vi "Experiment with Waveform Generation.vi"(6 "Default Values":T1={"X-Voltage (Default)"=10.0, "Y-Voltage (Default)"=10.0, "Pockels Voltage (Default)"=0.0, "GATE State (Default)"=FALSE}, 7 "Stim Points Array IN":T5[](array[typedef]), 8 "Trigger Parameters":T2, 9 "Sampling Rates":T3, 10 "Group Parameters":T4) -> (0 "Group Duration (Seconds)":dbl, 1 "Gate Wavefprm (digital)":digitalwaveform(waveform)={"t0"=timestamp(0 s since 1904-01-01), "dt"=1.0, "Y"={"transitions"=[], "data"=[]}}, 2 "XY Waveform":waveform(dbl)[](array[waveform]), 3 "Pockels Waveform":waveform(dbl), 4 "Total Protocol Time (s)":dbl, 5 "Stim Waveform Graph":waveform(dbl)[](array[waveform]))   [LabVIEW 2012]
uses:
  Custom Controls and Typedefs/Stim Waveform Parameters.ctl
  Custom Controls and Typedefs/GroupParameters_Cluster.ctl
  Custom Controls and Typedefs/SamplingRatesCluster.ctl
  Custom Controls and Typedefs/TriggerParameters_Cluster.ctl
  Custom Controls and Typedefs/SciScan System Information Cluster.ctl
  GFG/GFGbooleanGet.vi
  GFG/GFGstringGet.vi
  <vilib>/Waveform/DWDTOps.llb/DWDT Boolean Array to Digital.vi
  <vilib>/Utility/config.llb/Read Key (Double).vi
  GFG/GFGnumericGet.vi
  GFG/GFG library.lvlib
  <vilib>/Utility/config.llb/NI_LVConfig.lvlib
panel:
  out "error out":errorcluster
  in  "error in (no error)":errorcluster
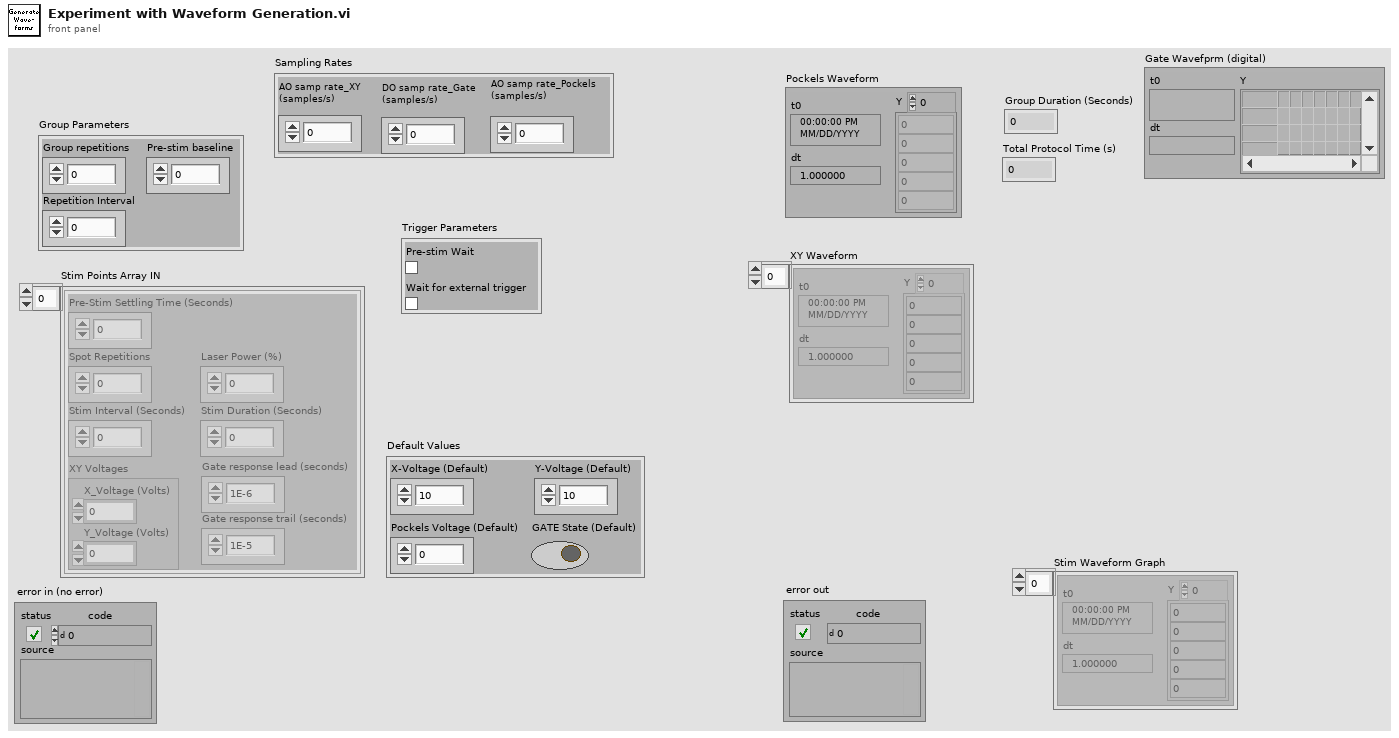
[diagram p1: front panel]
types:
  T1 = cluster{"X-Voltage (Default)":dbl, "Y-Voltage (Default)":dbl, "Pockels Voltage (Default)":dbl, "GATE State (Default)":bool}
  T2 = typedef "TriggerParameters_Cluster.ctl" = cluster{"Pre-stim Wait":bool, "Wait for external trigger":bool}
  T3 = typedef "SamplingRatesCluster.ctl" = cluster{"AO samp rate_XY (samples/s)":dbl, "AO samp rate_Pockels (samples/s)":dbl, "DO samp rate_Gate (samples/s)":dbl}
  T4 = typedef "GroupParameters_Cluster.ctl" = cluster{"Group repetitions":i32, "Repetition Interval":dbl, "Pre-stim baseline":dbl}
  T5 = typedef "Stim Waveform Parameters.ctl" = cluster{"Stim Interval (Seconds)":dbl, "Pre-Stim Settling Time (Seconds)":dbl, "Stim Duration (Seconds)":dbl, "Spot Repetitions":i32, "Laser Power (%)":dbl, "XY Voltages":cluster{"X_Voltage (Volts)":dbl, "Y_Voltage (Volts)":dbl}, "Gate response lead (seconds)":dbl, "Gate response trail (seconds)":dbl}
  T6 = typedef "SciScan System Information Cluster.ctl" = cluster{"Scanner Type":string, "Is it Hyperscope?":bool, "Hyperscope (DAQ) type":string}
  T7 = typedef "NI_LVConfig.lvlib/Config Data RefNum.ctl" = refnum<k1>
  T8 = cluster{"X_Voltage (Volts)":dbl, "Y_Voltage (Volts)":dbl}
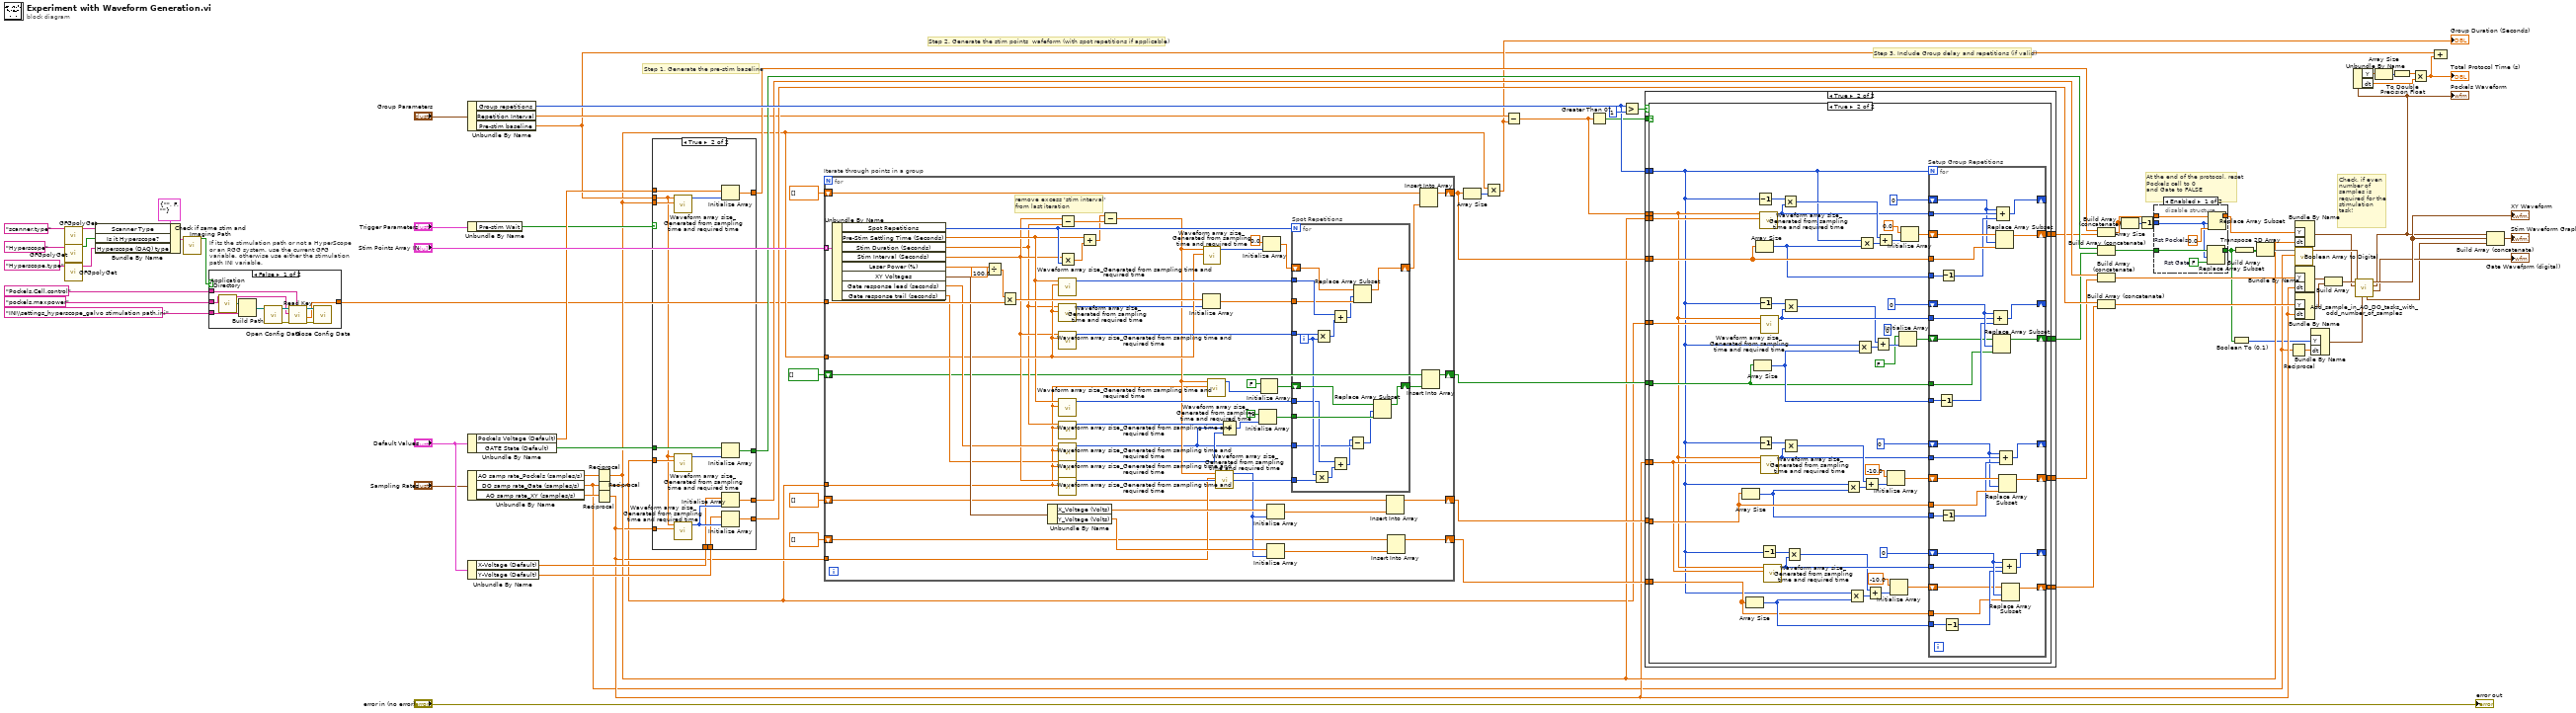
[diagram p0: block diagram]
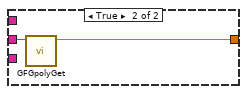
[diagram p3: hidden frame]
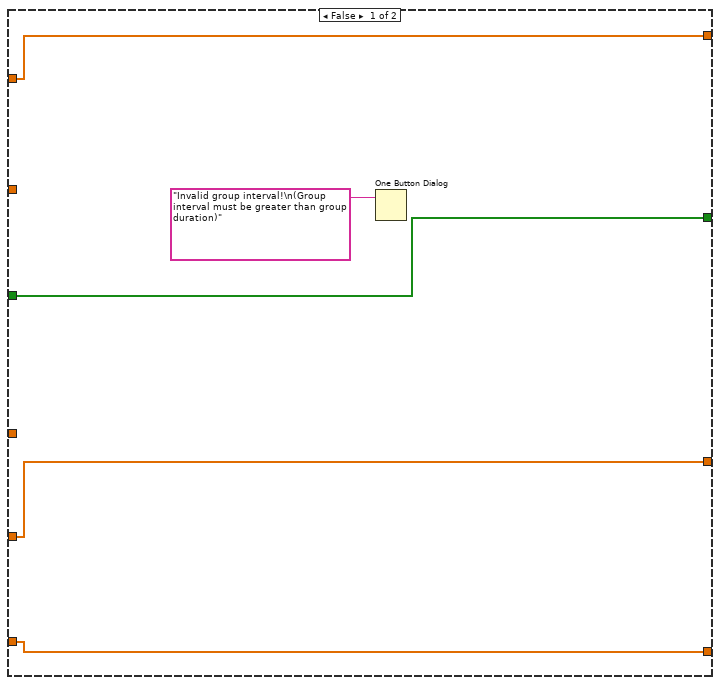
[diagram p6: hidden frame]
diagram:
  # "At the end of the protocol, reset Pockels cell to 0\nand Gate to FALSE"
  # "Check, if even number of samples is required for the stimulation task!"
  # "Step 1. Generate the pre-stim baseline"
  # "Step 3. Include Group delay and repetitions (if valid)"
  # "Step 2. Generate the stim points  wafeform (with spot repetitions if applicable)"
  n1 = call-poly "GFGpolyGet.vi"("Variable Name in"="scanner.type") -> ("String"=w19:string)  [unwired: 9 in, 1 out]
  n2 = call-poly "GFGpolyGet.vi"("Variable Name in"="Hyperscope") -> ("Boolean Value OUT"=w18:bool)  [unwired: 9 in, 1 out]
  n3 = call-poly "GFGpolyGet.vi"("Variable Name in"="Hyperscope.type") -> ("String"=w17:string)  [unwired: 9 in, 1 out]
  n4 = Bundle By Name(cluster=T6 {"Scanner Type"="", "Is it Hyperscope?"=FALSE, "Hyperscope (DAQ) type"=""} ("System Information Cluster"), "Scanner Type"=w19, "Is it Hyperscope?"=w18, "Hyperscope (DAQ) type"=w17) -> (w16:T6)
  n5 = call "Check if same stim and Imaging Path.vi"("System Information Cluster"=w16) -> ("Boolean"=w15:bool)  [unwired: 10 in]
  n6 = case "If its the stimulation path or not a HyperScope or an RGG system, use the current GFG variable, otherwise use either the stimulation path INI variable." shown="False" w15 {
    tunnel: [w84 w95] -> w24
    tunnel: "Pockels.Cell.control" ("Variable Name in") -> [w86 _]
    tunnel: "pockels.maxpower" ("name or relative path") -> [w85 w94]
    tunnel: "INI\\settings_hyperscope_galvo stimulation path.ini" ("name or relative path") -> [w87 _]
    frame False {
      n7 = call <vilib>:"Application Directory.vi"() -> ("Application Directory"=w88:path)
      n8 = Build Path(base path=w88, name or relative path=w87) -> (appended path=w89:path)
      n9 = call <vilib>:"Open Config Data.vi"("configuration file path"=w89) -> ("error out"=w93:errorcluster, "refnum"=w90:T7)  [unwired: 8 in, 1 out]
      n10 = call-poly <vilib>:"Read Key.vi"("section"=w86, "error in (no error)"=w93, "key"=w85, "refnum"=w90) -> ("error out"=w92:errorcluster, "value"=w84:dbl, "refnum out"=w91:T7)  [unwired: 4 in, 1 out]
      n11 = call <vilib>:"Close Config Data.vi"("error in (no error)"=w92, "refnum"=w91) -> ()  [unwired: 8 in, 2 out]
    }
    frame True {
      n12 = call-poly "GFGpolyGet.vi"("Variable Name in"=w94) -> ("Numeric"=w95:dbl)  [unwired: 8 in, 2 out]
    }
  }
  n13 = Unbundle By Name("Group Parameters") -> ("Group repetitions"=w77:i32, "Repetition Interval"=w48:dbl, "Pre-stim baseline"=w46:dbl)
  n14 = Unbundle By Name("Trigger Parameters") -> ("Pre-stim Wait"=w65:bool)
  n15 = Unbundle By Name("Default Values") -> ("Pockels Voltage (Default)"=w72:dbl, "GATE State (Default)"=w71:bool)
  n16 = Unbundle By Name("Sampling Rates") -> ("AO samp rate_Pockels (samples/s)"=w81:dbl, "DO samp rate_Gate (samples/s)"=w11:dbl, "AO samp rate_XY (samples/s)"=w80:dbl)
  n17 = Unbundle By Name("Default Values") -> ("X-Voltage (Default)"=w75:dbl, "Y-Voltage (Default)"=w74:dbl)
  n18 = Reciprocal(x=w81) -> (1/x=w37:dbl)
  n19 = Reciprocal(x=w11) -> (1/x=w35:dbl)
  n20 = Reciprocal(x=w80) -> (1/x=w36:dbl)
  n21 = case shown="True" w65 {
    tunnel: w36 -> [_ w110]
    tunnel: w35 -> [_ w109]
    tunnel: w37 -> [_ w108]
    tunnel: w75 -> [_ w104]
    tunnel: w74 -> [_ w103]
    tunnel: w72 -> [_ w102]
    tunnel: w71 -> [_ w101]
    tunnel: w46 -> [_ w100]
    tunnel: [_ w99] -> w59
    tunnel: [_ w98] -> w58
    tunnel: [_ w97] -> w57
    tunnel: [_ w96] -> w56
    frame False {
    }
    frame True {
      n22 = call "Waveform array size_Generated from sampling time and required time.vi"("Sample time in Seconds (dT = 1/Fs)"=w108, "Task time in seconds"=w100) -> ("Array Size OUT"=w107:i32)  [unwired: 9 in]
      n23 = call "Waveform array size_Generated from sampling time and required time.vi"("Sample time in Seconds (dT = 1/Fs)"=w109, "Task time in seconds"=w100) -> ("Array Size OUT"=w106:i32)  [unwired: 9 in]
      n24 = call "Waveform array size_Generated from sampling time and required time.vi"("Sample time in Seconds (dT = 1/Fs)"=w110, "Task time in seconds"=w100) -> ("Array Size OUT"=w105:i32)  [unwired: 9 in]
      n25 = Initialize Array(w102, w107) -> (w99:dbl[])
      n26 = Initialize Array(w101, w106) -> (w98:bool[])
      n27 = Initialize Array(w104, w105) -> (w97:dbl[])
      n28 = Initialize Array(w103, w105) -> (w96:dbl[])
    }
  }
  n29 = for "Iterate through points in a group" {
    tunnel: "Stim Points Array IN" -> [w163] mode=indexing
    tunnel: w37 -> [w147]
    tunnel: w24 -> [w161]
    tunnel: w35 -> [w114]
    tunnel: w36 -> [w138]
    shift-right: [w127] -> w60
    shift-left: dbl[] [] -> [w128]
    shift-right: [w124] -> w76
    shift-left: dbl[] [] -> [w125]
    shift-right: [w122] -> w70
    shift-left: bool[] [] -> [w111]
    shift-right: [w119] -> w62
    shift-left: dbl[] [] -> [w120]
    # "remove excess 'stim interval' from last iteration"
    n30 = Unbundle By Name(w163) -> ("Spot Repetitions"=w158:i32, "Pre-Stim Settling Time (Seconds)"=w141:dbl, "Stim Duration (Seconds)"=w132:dbl, "Stim Interval (Seconds)"=w133:dbl, "Laser Power (%)"=w136:dbl, "XY Voltages"=w153:T8, "Gate response lead (seconds)"=w148:dbl, "Gate response trail (seconds)"=w115:dbl)
    n31 = Divide(x=w136, y=100.0) -> (x/y=w134:dbl)
    n32 = Multiply(x=w134, y=w161) -> (x*y=w159:dbl)
    n33 = Unbundle By Name(w153) -> ("X_Voltage (Volts)"=w152:dbl, "Y_Voltage (Volts)"=w151:dbl)
    n34 = call "Waveform array size_Generated from sampling time and required time.vi"("Sample time in Seconds (dT = 1/Fs)"=w147, "Task time in seconds"=w141) -> ("Array Size OUT"=w156:i32)  [unwired: 9 in]
    n35 = call "Waveform array size_Generated from sampling time and required time.vi"("Sample time in Seconds (dT = 1/Fs)"=w147, "Task time in seconds"=w132) -> ("Array Size OUT"=w146:i32)  [unwired: 9 in]
    n36 = call "Waveform array size_Generated from sampling time and required time.vi"("Sample time in Seconds (dT = 1/Fs)"=w147, "Task time in seconds"=w133) -> ("Array Size OUT"=w157:i32)  [unwired: 9 in]
    n37 = call "Waveform array size_Generated from sampling time and required time.vi"("Sample time in Seconds (dT = 1/Fs)"=w114, "Task time in seconds"=w141) -> ("Array Size OUT"=w139:i32)  [unwired: 9 in]
    n38 = call "Waveform array size_Generated from sampling time and required time.vi"("Sample time in Seconds (dT = 1/Fs)"=w114, "Task time in seconds"=w132) -> ("Array Size OUT"=w142:i32)  [unwired: 9 in]
    n39 = call "Waveform array size_Generated from sampling time and required time.vi"("Sample time in Seconds (dT = 1/Fs)"=w114, "Task time in seconds"=w148) -> ("Array Size OUT"=w112:i32)  [unwired: 9 in]
    n40 = call "Waveform array size_Generated from sampling time and required time.vi"("Sample time in Seconds (dT = 1/Fs)"=w114, "Task time in seconds"=w115) -> ("Array Size OUT"=w113:i32)  [unwired: 9 in]
    n41 = call "Waveform array size_Generated from sampling time and required time.vi"("Sample time in Seconds (dT = 1/Fs)"=w114, "Task time in seconds"=w133) -> ("Array Size OUT"=w140:i32)  [unwired: 9 in]
    n42 = Subtract(x=w133, y=w132) -> (x-y=w131:dbl)
    n43 = Multiply(x=w133, y=w158) -> (x*y=w162:dbl)
    n44 = Add(x=w141, y=w162) -> (x+y=w130:dbl)
    n45 = Subtract(x=w130, y=w131) -> (x-y=w118:dbl)
    n46 = Initialize Array(w159, w146) -> (w155:dbl[])
    n47 = call "Waveform array size_Generated from sampling time and required time.vi"("Sample time in Seconds (dT = 1/Fs)"=w147, "Task time in seconds"=w118) -> ("Array Size OUT"=w150:i32)  [unwired: 9 in]
    n48 = call "Waveform array size_Generated from sampling time and required time.vi"("Sample time in Seconds (dT = 1/Fs)"=w114, "Task time in seconds"=w118) -> ("Array Size OUT"=w143:i32)  [unwired: 9 in]
    n49 = call "Waveform array size_Generated from sampling time and required time.vi"("Sample time in Seconds (dT = 1/Fs)"=w138, "Task time in seconds"=w118) -> ("Array Size OUT"=w137:i32)  [unwired: 9 in]
    n50 = Compound Arithmetic op=ADD(w142, w112, w113) -> (w145:i32)
    n51 = Initialize Array(TRUE, w145) -> (w144:bool[])
    n52 = Initialize Array(FALSE, w143) -> (w149:bool[])
    n53 = Initialize Array(0.0 ("1/x"), w150) -> (w154:dbl[])
    n54 = Initialize Array(w152, w137) -> (w126:dbl[])
    n55 = Initialize Array(w151, w137) -> (w129:dbl[])
    n56 = for "Spot Repetitions" {
      N: w158 -> [_]
      tunnel: w157 -> [w180]
      tunnel: w156 -> [w179]
      tunnel: w155 -> [w177]
      shift-right: [w175] -> w121
      shift-left: w154 -> [w178]
      shift-right: [w172] -> w123
      shift-left: w149 -> [w174]
      tunnel: w112 -> [w166]
      tunnel: w144 -> [w173]
      tunnel: w140 -> [w169]
      tunnel: w139 -> [w167]
      i -> [w170]
      n57 = Multiply(x=w170, y=w169) -> (x*y=w168:i32)
      n58 = Multiply(x=w180, y=w170) -> (x*y=w171:i32)
      n59 = Add(x=w179, y=w171) -> (x+y=w176:i32)
      n60 = Add(x=w167, y=w168) -> (x+y=w165:i32)
      n61 = Subtract(x=w165, y=w166) -> (x-y=w164:i32)
      n62 = Replace Array Subset(array=w178, new element=w177, index=w176) -> (w175:dbl[])
      n63 = Replace Array Subset(array=w174, new element=w173, index=w164) -> (w172:bool[])
    }
    n64 = Insert Into Array(array=w125, new element=w126) -> (w124:dbl[])  [unwired: 1 in]
    n65 = Insert Into Array(array=w128, new element=w129) -> (w127:dbl[])  [unwired: 1 in]
    n66 = Insert Into Array(array=w120, new element=w121) -> (w119:dbl[])  [unwired: 1 in]
    n67 = Insert Into Array(array=w111, new element=w123) -> (w122:bool[])  [unwired: 1 in]
  }
  n68 = Array Size(array=w62) -> (size(s)=w61:i32)
  n69 = Multiply(x=w37, y=w61) -> (x*y=w47:dbl)
  "Group Duration (Seconds)" <- w47
  n70 = Subtract(x=w48, y=w47) -> (x-y=w63:dbl)
  n71 = Greater Than 0?(x=w63) -> (x > 0?=w64:bool)
  n72 = Greater?(x=w77, y=1) -> (0:w79:bool)
  n73 = case shown="True" w79 {
    tunnel: w62 -> [w184 w198]
    tunnel: w77 -> [_ w192]
    tunnel: w63 -> [_ w191]
    tunnel: w37 -> [_ w197]
    tunnel: w70 -> [w183 w196]
    tunnel: w35 -> [_ w195]
    tunnel: w76 -> [w182 w193]
    tunnel: w36 -> [_ w194]
    tunnel: w64 -> [_ w190]
    tunnel: [w184 w189] -> w55
    tunnel: [w183 w188] -> w54
    tunnel: w60 -> [w181 w187]
    tunnel: [w182 w186] -> w53
    tunnel: [w181 w185] -> w52
    frame False {
    }
    frame True {
      n74 = case shown="True" w190 {
        tunnel: w198 -> [w202 w250]
        tunnel: w197 -> [_ w249]
        tunnel: w196 -> [w201 w233]
        tunnel: w195 -> [_ w232]
        tunnel: w194 -> [_ w209]
        tunnel: w193 -> [w200 w231]
        tunnel: w192 -> [_ w207]
        tunnel: w191 -> [_ w208]
        tunnel: [w202 w221] -> w189
        tunnel: [w201 w220] -> w188
        tunnel: w187 -> [w199 w210]
        tunnel: [w200 w206] -> w186
        tunnel: [w199 w205] -> w185
        frame False {
          n75 = One Button Dialog(message="Invalid group interval!\n(Group interval must be greater than group duration)") -> ()  [unwired: 1 in, 1 out]
        }
        frame True {
          (unwired) u32 0 ("element")
          n76 = Array Size(array=w231) -> (size(s)=w222:i32)
          n77 = Array Size(array=w210) -> (size(s)=w219:i32)
          n78 = Array Size(array=w233) -> (size(s)=w241:i32)
          n79 = Array Size(array=w250) -> (size(s)=w242:i32)
          n80 = Decrement(x=w207) -> (x-1=w248:i32)
          n81 = Decrement(x=w207) -> (x-1=w235:i32)
          n82 = Decrement(x=w207) -> (x-1=w228:i32)
          n83 = call "Waveform array size_Generated from sampling time and required time.vi"("Sample time in Seconds (dT = 1/Fs)"=w249, "Task time in seconds"=w208) -> ("Array Size OUT"=w244:i32)  [unwired: 9 in]
          n84 = call "Waveform array size_Generated from sampling time and required time.vi"("Sample time in Seconds (dT = 1/Fs)"=w232, "Task time in seconds"=w208) -> ("Array Size OUT"=w239:i32)  [unwired: 9 in]
          n85 = call "Waveform array size_Generated from sampling time and required time.vi"("Sample time in Seconds (dT = 1/Fs)"=w209, "Task time in seconds"=w208) -> ("Array Size OUT"=w224:i32)  [unwired: 9 in]
          n86 = Decrement(x=w207) -> (x-1=w213:i32)
          n87 = call "Waveform array size_Generated from sampling time and required time.vi"("Sample time in Seconds (dT = 1/Fs)"=w209, "Task time in seconds"=w208) -> ("Array Size OUT"=w217:i32)  [unwired: 9 in]
          n88 = Multiply(x=w248, y=w244) -> (x*y=w246:i32)
          n89 = Multiply(x=w235, y=w239) -> (x*y=w237:i32)
          n90 = Multiply(x=w228, y=w224) -> (x*y=w226:i32)
          n91 = Multiply(x=w213, y=w217) -> (x*y=w215:i32)
          n92 = Multiply(x=w207, y=w222) -> (x*y=w227:i32)
          n93 = Multiply(x=w207, y=w219) -> (x*y=w214:i32)
          n94 = Multiply(x=w207, y=w241) -> (x*y=w236:i32)
          n95 = Multiply(x=w207, y=w242) -> (x*y=w247:i32)
          n96 = Add(x=w226, y=w227) -> (x+y=w225:i32)
          n97 = Add(x=w215, y=w214) -> (x+y=w216:i32)
          n98 = Add(x=w237, y=w236) -> (x+y=w238:i32)
          n99 = Add(x=w246, y=w247) -> (x+y=w245:i32)
          n100 = Initialize Array(-10.0 ("element"), w225) -> (w229:dbl[])
          n101 = Initialize Array(-10.0 ("element"), w216) -> (w212:dbl[])
          n102 = Initialize Array(FALSE, w238) -> (w234:bool[])
          n103 = Initialize Array(0.0 ("element"), w245) -> (w251:dbl[])
          n104 = for "Setup Group Repetitions" {
            N: w207 -> [_]
            tunnel: w250 -> [w283]
            shift-right: [w277] -> w221
            shift-left: w251 -> [w284]
            tunnel: w244 -> [w280]
            shift-right: [w278] -> _
            shift-left: 0 ("Array Size OUT") -> [w279]
            tunnel: w242 -> [w282]
            tunnel: w233 -> [w270]
            shift-right: [w276] -> w220
            shift-left: w234 -> [w269]
            tunnel: w239 -> [w273]
            shift-right: [w275] -> _
            shift-left: 0 ("Array Size OUT") -> [w274]
            tunnel: w241 -> [w271]
            tunnel: w231 -> [w267]
            shift-right: [w261] -> w206
            shift-left: w229 -> [w268]
            tunnel: w224 -> [w264]
            shift-right: [w262] -> _
            shift-left: 0 ("Array Size OUT") -> [w263]
            tunnel: w222 -> [w266]
            tunnel: w210 -> [w254]
            shift-right: [w260] -> w205
            shift-left: w212 -> [w253]
            tunnel: w217 -> [w257]
            shift-right: [w259] -> _
            shift-left: 0 ("Array Size OUT") -> [w258]
            tunnel: w219 -> [w255]
            n105 = Decrement(x=w271) -> (x-1=w272:i32)
            n106 = Decrement(x=w282) -> (x-1=w281:i32)
            n107 = Decrement(x=w266) -> (x-1=w265:i32)
            n108 = Decrement(x=w255) -> (x-1=w256:i32)
            n109 = Replace Array Subset(array=w269, new element=w270, index=w274) -> (w276:bool[])
            n110 = Compound Arithmetic op=ADD(w274, w273, w272) -> (w275:i32)
            n111 = Replace Array Subset(array=w284, new element=w283, index=w279) -> (w277:dbl[])
            n112 = Compound Arithmetic op=ADD(w279, w280, w281) -> (w278:i32)
            n113 = Replace Array Subset(array=w268, new element=w267, index=w263) -> (w261:dbl[])
            n114 = Compound Arithmetic op=ADD(w263, w264, w265) -> (w262:i32)
            n115 = Replace Array Subset(array=w253, new element=w254, index=w258) -> (w260:dbl[])
            n116 = Compound Arithmetic op=ADD(w258, w257, w256) -> (w259:i32)
          }
        }
      }
    }
  }
  n117 = Build Array (concatenate)(w59, w55) -> (w5:dbl[])
  n118 = Build Array (concatenate)(w58, w54) -> (w3:bool[])
  n119 = Build Array (concatenate)(w57, w53) -> (w50:dbl[])
  n120 = Build Array (concatenate)(w56, w52) -> (w49:dbl[])
  n121 = Array Size(array=w5) -> (size(s)=w6:i32)
  n122 = Decrement(x=w6) -> (x-1=w1:i32)
  n123 = disable-structure shown="Enabled" {
    disable-tunnel: w5 -> [w291 w293]
    disable-tunnel: [w290 w293] -> w4
    disable-tunnel: w3 -> [w288 w292]
    disable-tunnel: [w287 w292] -> w2
    disable-tunnel: w1 -> [w286 _]
    frame Enabled {
      w285 = FALSE  # Rst Gate
      w289 = 0.0  # Rst Pockels
      n124 = Replace Array Subset(array=w288, new element=w285, index=w286) -> (w287:bool[])
      n125 = Replace Array Subset(array=w291, new element=w289, index=w286) -> (w290:dbl[])
    }
    frame Disabled {
    }
  }
  n126 = Boolean To (0,1)(Boolean=w2) -> (0, 1=w9:i16[])
  n127 = Build Array(w2) -> (w40:bool[][])
  n128 = Transpose 2D Array(2D array=w40) -> (transposed array=w39:bool[][])
  n129 = Reciprocal(x=w11) -> (1/x=w10:dbl)
  n130 = Bundle By Name("Y"=w4, "dt"=w37) -> (w26:waveform(dbl))  [unwired: 1 in]
  n131 = call-poly <vilib>:"Boolean Array to Digital.vi"("sample rate"=w11, "boolean array"=w39) -> ("digital waveform"=w28:digitalwaveform)  [unwired: 8 in, 1 out]
  n132 = Bundle By Name("Y"=w50, "dt"=w36) -> (w41:waveform(dbl))  [unwired: 1 in]
  n133 = Bundle By Name("Y"=w49, "dt"=w36) -> (w42:waveform(dbl))  [unwired: 1 in]
  n134 = Bundle By Name("Y"=w9, "dt"=w10) -> (w8:waveform(i16))  [unwired: 1 in]
  n135 = Build Array(w41, w42) -> (w30:waveform(dbl)[])
  n136 = call "Add_sample_in_AO_DO_tasks_with_odd_number_of_samples.vi"("Dummy Gate Waveform IN"=w8, "Gate Waveform (Digital) IN"=w28, "Pockels Waveform IN"=w26, "XY Waveform IN"=w30) -> ("Gate Waveform (Digital) OUT"=→"Gate Wavefprm (digital)":digitalwaveform, "Pockels Waveform OUT"=w25:waveform(dbl), "XY Waveform OUT"=w29:waveform(dbl)[], "Dummy Gate Waveform OUT"=w7:waveform(i16))  [unwired: 2 in, 2 out]
  "XY Waveform" <- w29
  "Pockels Waveform" <- w25
  n137 = Unbundle By Name(w25) -> ("Y"=w34:dbl[], "dt"=w31:dbl)
  n138 = Array Size(array=w34) -> (size(s)=w33:i32)
  n139 = To Double Precision Float(number=w33) -> (double precision float=w32:dbl)
  n140 = Multiply(x=w32, y=w31) -> (x*y=w45:dbl)
  "Total Protocol Time (s)" <- w45
  n141 = Compound Arithmetic op=ADD(w46, w45) -> ()  [unwired: 1 out]
  n142 = Build Array (concatenate)(w25, w29, w7) -> (→"Stim Waveform Graph":waveform(dbl)[])
  "error out" <- "error in (no error)"
